vi "FTW-Request-Deserialize.vi"(0 "Message":string, 11 "error in":errorcluster) -> (4 "Message Header":string, 6 "Message Body":string, 15 "error out":errorcluster)   [LabVIEW 2013, in "FTW-Request.lvclass"]
uses:
  FTW-Request.lvclass
  error/FTW-ERR-ExceptionType.ctl
  error/FTW-ERR-NoErrorConstant.vi
  reflection/FTW-Reflection-Type.vi
  json/lib/FTW-JSON-Core-LibraryFilepath.vi
  json/lib/FTW-JSON-Core-GetFlattenedValue.vi
  json/lib/FTW-JSON-Core-LibraryError.vi
  error/FTW-ERR-CallChain.vi
  string/FTW-STR-ReplaceWhitespace.vi
  json/FTW-JSON-Deserialize/FTW-JSON-Deserialize.xnode
panel:
  # "Inputs"
  # "Outputs"
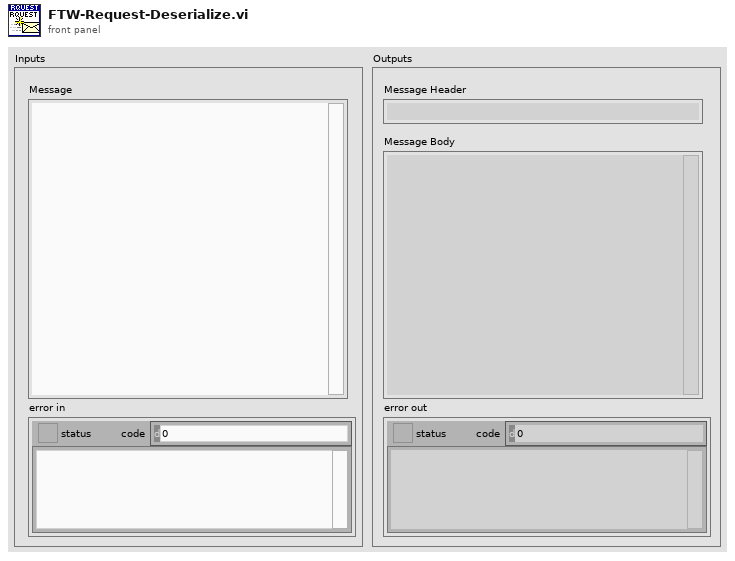
[diagram p1: front panel]
types:
  T1 = cluster{"Header":string, "Body":string, "ExceptionString":string, "ExceptionType":string, "ExceptionCode":i32}
  T2 = typedef "FTW-ERR-ExceptionType.ctl" = enum16{"OK", "Error", "Warning"}
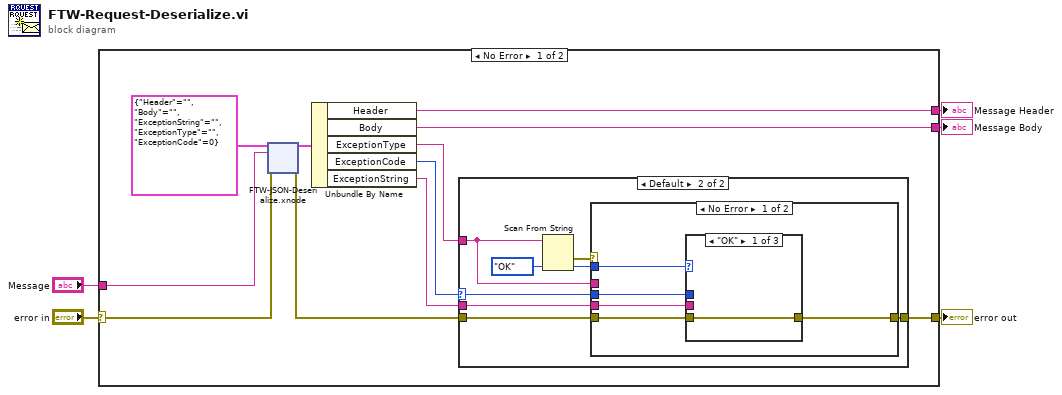
[diagram p0: block diagram]
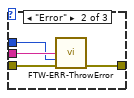
[diagram p3: hidden frame]
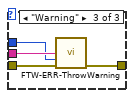
[diagram p4: hidden frame]
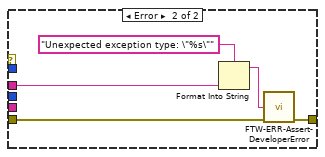
[diagram p5: hidden frame]
diagram:
  n1 = case shown="No Error" "error in" {
    selector: "error in" -> [w15 w79]
    tunnel: [w9 w79] -> w5
    tunnel: "Message" -> [w16 _]
    tunnel: [w12 _] -> w2
    tunnel: [w11 _] -> w1
    frame No Error {
      n2 = xnode "FTW-JSON-Deserialize.xnode"("Type and Defaults"=T1 {"Header"="", "Body"="", "ExceptionString"="", "ExceptionType"="", "ExceptionCode"=0}, "JSON String"=w16, "error in"=w15) -> ("Values"=w13:T1, "error out"=w10:errorcluster)
      n3 = Unbundle By Name(w13) -> ("Header"=w12:string, "Body"=w11:string, "ExceptionType"=w8:string, "ExceptionCode"=w6:i32, "ExceptionString"=w7:string)
      n4 = case shown="Default" w6 {
        selector: w6 -> [_ w18]
        tunnel: w10 -> [w17 w23]
        tunnel: [w17 w22] -> w9
        tunnel: w8 -> [_ w21]
        tunnel: w7 -> [_ w19]
        frame 0 {
        }
        frame Default {
          n5 = Scan From String(input string=w21, default 1=FTW-ERR-ExceptionType."OK" ("Exception")) -> (error out=w24:errorcluster, output 1=w20:T2)  [unwired: 3 in, 2 out]
          n6 = case shown="No Error" w24 {
            tunnel: w23 -> [w28 w44]
            tunnel: [w29 w43] -> w22
            tunnel: w21 -> [_ w40]
            tunnel: w20 -> [w30 _]
            tunnel: w18 -> [w26 _]
            tunnel: w19 -> [w27 _]
            frame No Error {
              n7 = case shown="\"OK\"" w30 {
                tunnel: [w31 w34 w38] -> w29
                tunnel: w28 -> [w31 w35 w39]
                tunnel: w27 -> [_ w33 w37]
                tunnel: w26 -> [_ w32 w36]
                frame "OK" {
                }
                frame "Error" {
                  n8 = call "FTW-ERR-ThrowError.vi"("Error Message"=w33, "Error Code"=w32, "error in"=w35) -> ("error out"=w34:errorcluster)  [unwired: 12 in]
                }
                frame "Warning" {
                  n9 = call "FTW-ERR-ThrowWarning.vi"("Warning Message"=w37, "Warning Code"=w36, "error in"=w39) -> ("error out"=w38:errorcluster)  [unwired: 12 in]
                }
              }
            }
            frame Error {
              n10 = Format Into String(format string="Unexpected exception type: \"%s\"", w40) -> (resulting string=w41:string)  [unwired: 2 in, 1 out]
              n11 = call "FTW-ERR-Assert-DeveloperError.vi"("Reason this error should never happen"=w41, "error in"=w44) -> ("error out"=w43:errorcluster)  [unwired: 13 in]
            }
          }
        }
      }
    }
    frame Error {
    }
  }
  "error out" <- w5
  "Message Header" <- w2
  "Message Body" <- w1
